vi "LickPortPosfilter.vi"(3 "audio off state (V)":dbl, 4 "audio filter period(uSec)":i32, 5 "audio threshold":fxp<+/-,16,5>, 6 "input":dbl) -> (2 "output":bool)   [LabVIEW 2014]
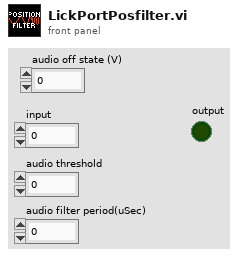
[diagram p1: front panel]
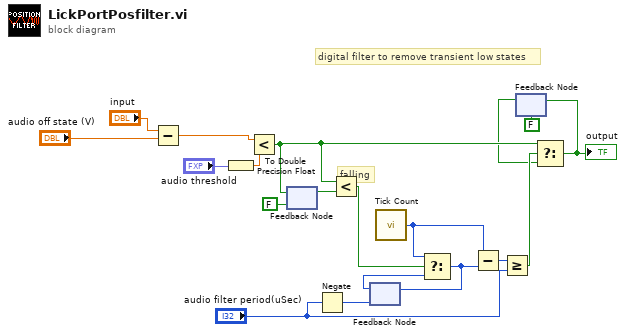
[diagram p0: block diagram]
diagram:
  # "digital filter to remove transient low states"
  # "falling"
  n1 = Subtract(x="input", y="audio off state (V)") -> (x-y=w1:dbl)
  n2 = To Double Precision Float(number="audio threshold") -> (double precision float=w4:dbl)
  n3 = Less?(x=w1, y=w4) -> (x < y?=w15:bool)
  n4 = feedback #1(FALSE) -> (w14:bool)
  n5 = feedback-in #1(w15) -> ()
  n6 = Negate(x="audio filter period(uSec)") -> (-x=w9:i32)
  n7 = Less?(x=w15, y=w14) -> (x < y?=w19:bool)
  n8 = feedback #2(w9) -> (w11:u32)
  n9 = call "Tick Count"() -> ("Tick Count(uSec)"=w18:u32)
  n10 = Select(t=w18, s=w19, f=w11) -> (s? t:f=w12:u32)
  n11 = feedback-in #2(w12) -> ()
  n12 = Subtract(x=w18, y=w12) -> (x-y=w17:u32)
  n13 = Greater Or Equal?(x=w17, y="audio filter period(uSec)") -> (x >= y?=w16:bool)
  n14 = feedback #3(FALSE) -> (w7:bool)
  n15 = Select(t=w15, s=w16, f=w7) -> (s? t:f=w8:bool)
  "output" <- w8
  n16 = feedback-in #3(w8) -> ()
